vi "MISC Update Test End Time.vi"(0 "Data File":string) -> (4 "New Data File":string)   [LabVIEW 2011]
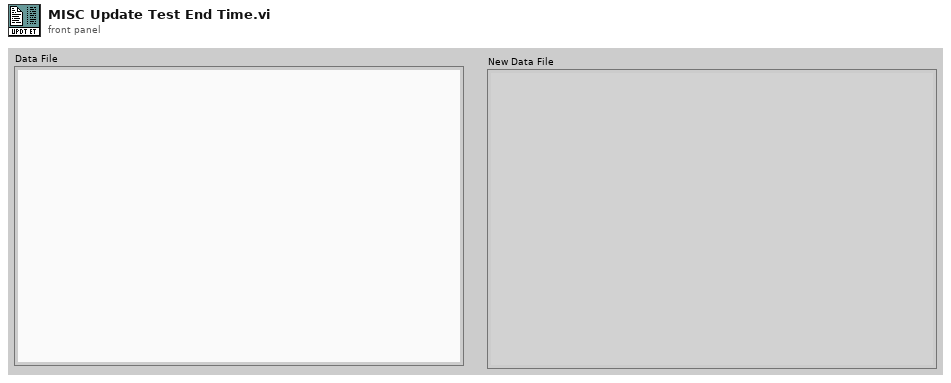
[diagram p1: front panel]
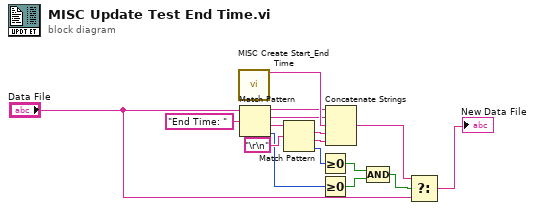
[diagram p0: block diagram]
diagram:
  n1 = call "MISC Create Start_End Time.vi"() -> ("Time"=w11:string)  [unwired: 14 in, 1 out]
  n2 = Match Pattern(string="Data File", regular expression="End Time: " ("Search Text")) -> (before substring=w10:string, match substring=w9:string, after substring=w15:string, offset past match=w5:i32)  [unwired: 1 in]
  n3 = Match Pattern(string=w15, regular expression="\r\n") -> (match substring=w12:string, after substring=w13:string, offset past match=w4:i32)  [unwired: 1 in, 1 out]
  n4 = Greater Or Equal To 0?(x=w4) -> (x >= 0?=w8:bool)
  n5 = Greater Or Equal To 0?(x=w5) -> (x >= 0?=w7:bool)
  n6 = Concatenate Strings(w10, w9, w11, w12, w13) -> (w2:string)
  n7 = Compound Arithmetic op=AND(w8, w7) -> (w3:bool)
  n8 = Select(t=w2, s=w3, f="Data File") -> (s? t:f=→"New Data File":string)
